vi "Dispense FN - OFF (SubVI).vi"(0 "Signals IN":T2={"Dispense"=FALSE, "Fill"=FALSE, "Spray"=FALSE, "Drain"=TRUE, "Complete"=FALSE, "Fill Error"=FALSE, "Dispense Error"=FALSE, "Fill Timeout"=FALSE, "Dispense Timeout"=FALSE}, 1 "Values IN":T3 {"Time Elapsed (s)" format="%.2f"; "Time Target (s)" format="%.2f"; "Dynamic Setpoint (g)" format="%.2f"; "Static Setpoint (g)" format="%.2f"; "Grams to Setpoint" format="%.2f"; "Adjusted Mass (g)" format="%.2f"; "Dispense Rate (g/sec)" format="%.2f"; "Fill Mass (g)" format="%.2f"; "Fill Rate (g/sec)" format="%.2f"}, 2 "Settings":T1={"ON Settings"={"Enable Dynamic Setpoint?"=TRUE, "Enable Dynamic Dispense Time?"=TRUE, "Enable Drain Rate Functions"=TRUE, "Dispense Sample Time (s)"=0.5, "Dispense Slope Ave"=0, "ON Timeout (sec)"=600.0, "1st Setpoint (% of Target)"=0.0, "2nd Setpoint (% of Target)"=0.0, "3rd Setpoint (% of Target)"=0.0, "Measure Dispense Delay (sec)"=0.0, "Settle Slope Sample Time (s)"=0.0}, "OFF Settings"={"Drain Sample Time (s)"=0.5, "Drain Rate Ave Size"=5, "Drain Rate Limits (± g/sec)"=10.0, "Level Slope Range (± g/sec)"=0.25, "OFF Timeout (sec)"=0.0, "Near SP Slope Level (± g/sec)"=0.01, "Near Setpoint Threshold (%)"=95.0}, "Overshoot Settings"={"Time Limit (s)"=60.0, "Container MAX (g)"=1500.0, "Max FILL Slope (+/- g/sec)"=10.0, "% Overshot to Enable (>)"=0.25}, "FILL Timeout (s)"=300.0, "Full Settle Time (s)"=3.0, "Pre-Hydrate \nSpray Time (s)"=10.0, "Pre-Hydrate \nWait Time (s)"=30.0}, 3 "Measured Mass (g)":dbl, 5 "State Change?":bool) -> (14 "Signals OUT":T2={"Dispense"=FALSE, "Fill"=FALSE, "Spray"=FALSE, "Drain"=TRUE, "Complete"=FALSE, "Fill Error"=FALSE, "Dispense Error"=FALSE, "Fill Timeout"=FALSE, "Dispense Timeout"=FALSE}, 15 "Values OUT":T3 {"Time Elapsed (s)" format="%.2f"; "Time Target (s)" format="%.2f"; "Dynamic Setpoint (g)" format="%.2f"; "Static Setpoint (g)" format="%.2f"; "Grams to Setpoint" format="%.2f"; "Adjusted Mass (g)" format="%.2f"; "Dispense Rate (g/sec)" format="%.2f"; "Fill Mass (g)" format="%.2f"; "Fill Rate (g/sec)" format="%.2f"}, 19 "ON Signal":bool)   [LabVIEW 2012]
panel:
  out "Level Slope?":bool
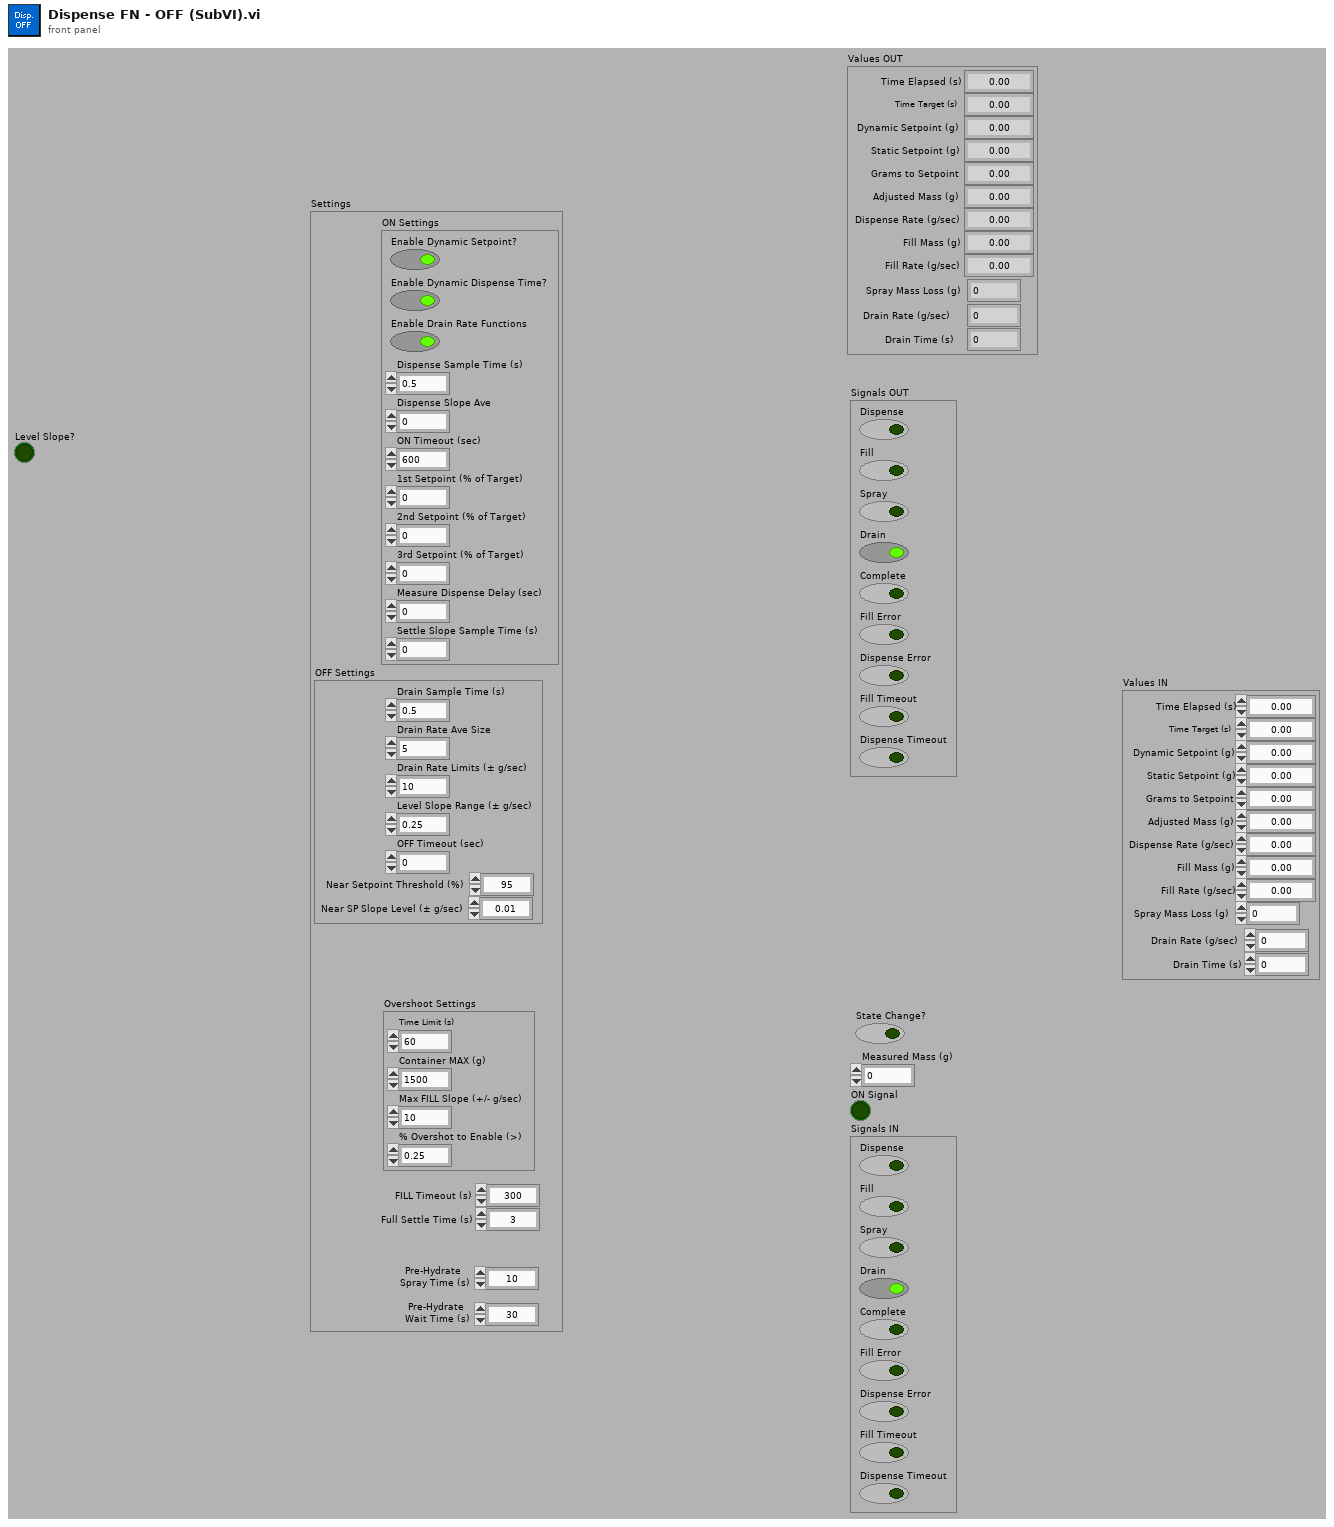
[diagram p1: front panel]
types:
  T1 = cluster{"ON Settings":cluster{"Enable Dynamic Setpoint?":bool, "Enable Dynamic Dispense Time?":bool, "Enable Drain Rate Functions":bool, "Dispense Sample Time (s)":dbl, "Dispense Slope Ave":i32, "ON Timeout (sec)":dbl, "1st Setpoint (% of Target)":dbl, "2nd Setpoint (% of Target)":dbl, "3rd Setpoint (% of Target)":dbl, "Measure Dispense Delay (sec)":dbl, "Settle Slope Sample Time (s)":dbl}, "OFF Settings":cluster{"Drain Sample Time (s)":dbl, "Drain Rate Ave Size":i32, "Drain Rate Limits (± g/sec)":dbl, "Level Slope Range (± g/sec)":dbl, "OFF Timeout (sec)":dbl, "Near SP Slope Level (± g/sec)":dbl, "Near Setpoint Threshold (%)":dbl}, "Overshoot Settings":cluster{"Time Limit (s)":dbl, "Container MAX (g)":dbl, "Max FILL Slope (+/- g/sec)":dbl, "% Overshot to Enable (>)":dbl}, "FILL Timeout (s)":dbl, "Full Settle Time (s)":dbl, "Pre-Hydrate \nSpray Time (s)":dbl, "Pre-Hydrate \nWait Time (s)":dbl}
  T2 = cluster{"Dispense":bool, "Fill":bool, "Spray":bool, "Drain":bool, "Complete":bool, "Fill Error":bool, "Dispense Error":bool, "Fill Timeout":bool, "Dispense Timeout":bool}
  T3 = cluster{"Time Elapsed (s)":dbl, "Time Target (s)":dbl, "Dynamic Setpoint (g)":dbl, "Static Setpoint (g)":dbl, "Grams to Setpoint":dbl, "Adjusted Mass (g)":dbl, "Dispense Rate (g/sec)":dbl, "Fill Mass (g)":dbl, "Fill Rate (g/sec)":dbl, "Spray Mass Loss (g)":dbl, "Drain Rate (g/sec)":dbl, "Drain Time (s)":dbl}
  T4 = cluster{"Settled Slope UL":dbl, "Settled Slope LL":dbl, "OFF Timeout (sec)":dbl, "Settle Slope Ave":i32, "Dispense Slope Ave":i32, "ON Timeout (sec)":dbl, "Dispense Slope Sample Time (s)":dbl, "1st Setpoint (% of Target)":dbl, "2nd Setpoint (% of Target)":dbl, "3rd Setpoint (% of Target)":dbl, "Enable Dynamic Setpoint?":bool, "Enable Dynamic Dispense Time?":bool, "Measure Dispense Delay (sec)":dbl, "Settle Slope Sample Time (s)":dbl}
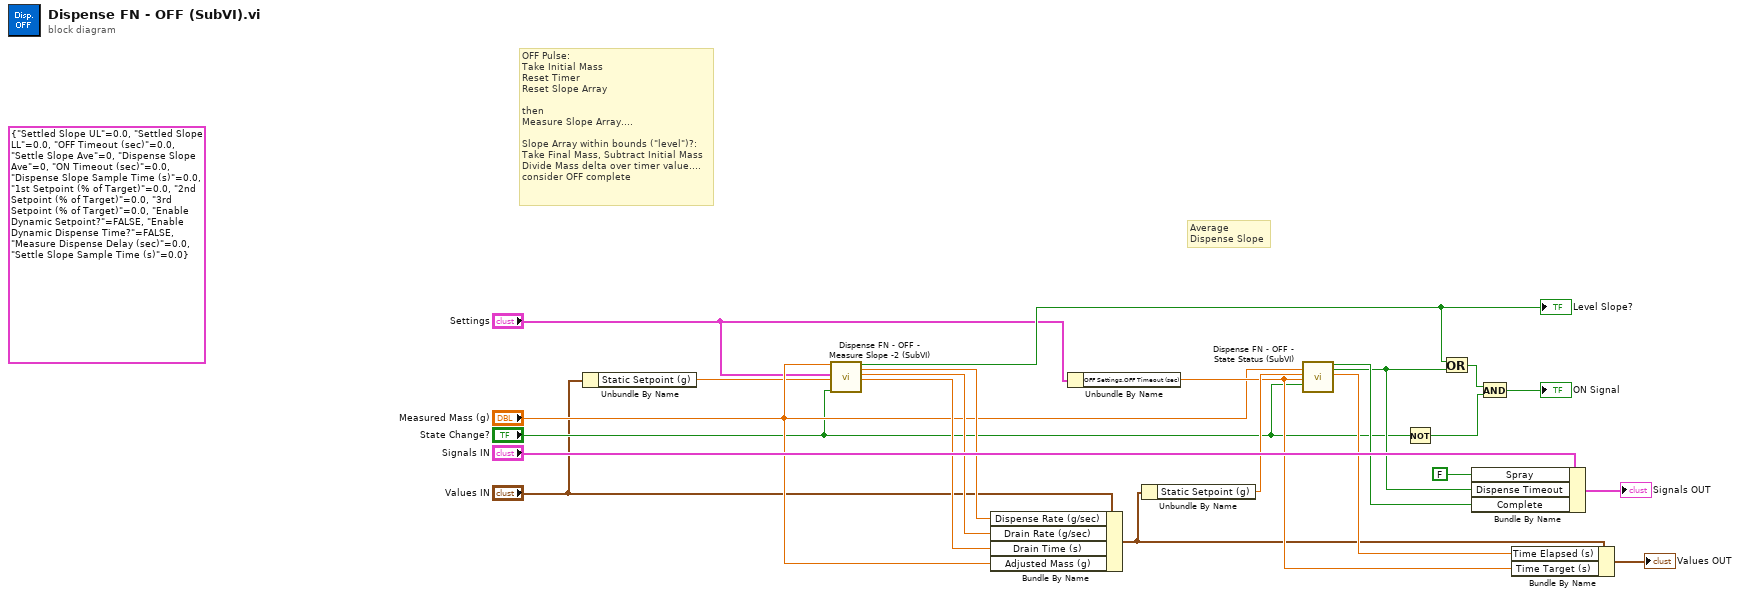
[diagram p0: block diagram]
diagram:
  (unwired) T4 {"Settled Slope UL"=0.0, "Settled Slope LL"=0.0, "OFF Timeout (sec)"=0.0, "Settle Slope Ave"=0, "Dispense Slope Ave"=0, "ON Timeout (sec)"=0.0, "Dispense Slope Sample Time (s)"=0.0, "1st Setpoint (% of Target)"=0.0, "2nd Setpoint (% of Target)"=0.0, "3rd Setpoint (% of Target)"=0.0, "Enable Dynamic Setpoint?"=FALSE, "Enable Dynamic Dispense Time?"=FALSE, "Measure Dispense Delay (sec)"=0.0, "Settle Slope Sample Time (s)"=0.0} ("Settings 2")
  # "OFF Pulse:\nTake Initial Mass\nReset Timer\nReset Slope Array\n\nthen\nMeasure Slope Array....\n\nSlope Array within bounds (\"level\")?:\nTake Final Mass, Subtract Initial Mass\nDivide Mass delta over timer value....\nconsider OFF complete"
  # "Average\nDispense Slope"
  n1 = Unbundle By Name("Values IN") -> ("Static Setpoint (g)"=w3:dbl)
  n2 = call "Dispense FN - OFF - Measure Slope -2 (SubVI).vi"("Measured Mass (g)"="Measured Mass (g)", "Settings"="Settings", "Static Setpoint (g)"=w3, "Initialize"="State Change?") -> ("Level Signal"=w12:bool, "Ave. Slope (g/sec)"=w15:dbl, "Rate (g/sec)"=w19:dbl, "Time (s)"=w18:dbl)  [unwired: 12 out]
  "Level Slope?" <- w12
  n3 = Bundle By Name(cluster="Values IN", "Dispense Rate (g/sec)"=w15, "Drain Rate (g/sec)"=w19, "Drain Time (s)"=w18, "Adjusted Mass (g)"="Measured Mass (g)") -> (w1:T3)
  n4 = Unbundle By Name("Settings") -> ("OFF Settings.OFF Timeout (sec)"=w13:dbl)
  n5 = Unbundle By Name(w1) -> ("Static Setpoint (g)"=w17:dbl)
  n6 = call "Dispense FN - OFF - State Status (SubVI).vi"("Measured Mass (g)"="Measured Mass (g)", "Static Setpoint (g)"=w17, "Timeout (s)"=w13, "State Change Pulse"="State Change?") -> ("Complete"=w14:bool, "Timed Out"=w11:bool, "Time Elapsed (s)"=w16:dbl)  [unwired: 13 out]
  n7 = Not(x="State Change?") -> (.not. x?=w8:bool)
  n8 = Or(x=w12, y=w11) -> (x .or. y?=w7:bool)
  n9 = Bundle By Name(cluster="Signals IN", "Spray"=FALSE, "Dispense Timeout"=w11, "Complete"=w14) -> (→"Signals OUT":T2)
  n10 = And(x=w7, y=w8) -> (x .and. y?=→"ON Signal":bool)
  n11 = Bundle By Name(cluster=w1, "Time Elapsed (s)"=w16, "Time Target (s)"=w13) -> (→"Values OUT":T3)
